vi "Snake.vi"(10 "Snake":dbl, 11 "Crab Degree":dbl) -> (0 "FR":dbl, 1 "FL":dbl, 2 "RR":dbl, 3 "RL":dbl)   [LabVIEW 2016]
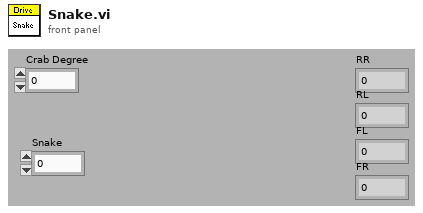
[diagram p1: front panel]
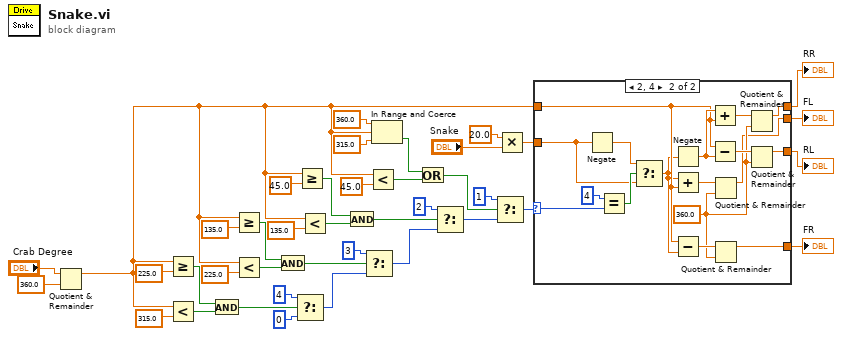
[diagram p0: block diagram]
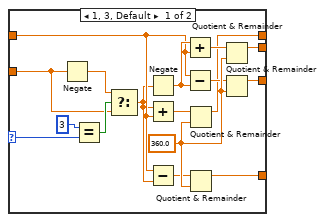
[diagram p2: hidden frame]
diagram:
  n1 = Quotient & Remainder(x="Crab Degree", y=360.0) -> (x-y*floor(x/y)=w1:dbl)  [unwired: 1 out]
  n2 = Greater Or Equal?(x=w1, y=225.0) -> (x >= y?=w18:bool)
  n3 = Less?(x=w1, y=315.0) -> (x < y?=w19:bool)
  n4 = And(x=w18, y=w19) -> (x .and. y?=w17:bool)
  n5 = Greater Or Equal?(x=w1, y=135.0) -> (x >= y?=w25:bool)
  n6 = Less?(x=w1, y=225.0) -> (x < y?=w24:bool)
  n7 = And(x=w25, y=w24) -> (x .and. y?=w11:bool)
  n8 = Select(t=4, s=w17, f=0) -> (s? t:f=w16:i32)
  n9 = Greater Or Equal?(x=w1, y=45.0) -> (x >= y?=w26:bool)
  n10 = Less?(x=w1, y=135.0) -> (x < y?=w27:bool)
  n11 = And(x=w26, y=w27) -> (x .and. y?=w12:bool)
  n12 = Select(t=3, s=w11, f=w16) -> (s? t:f=w15:i32)
  n13 = Less?(x=w1, y=45.0) -> (x < y?=w31:bool)
  n14 = In Range and Coerce(upper limit=360.0, x=w1, lower limit=315.0) -> (In Range?=w30:bool)  [unwired: 1 out]
  n15 = Or(x=w30, y=w31) -> (x .or. y?=w13:bool)
  n16 = Select(t=2, s=w12, f=w15) -> (s? t:f=w14:i32)
  n17 = Select(t=1, s=w13, f=w14) -> (s? t:f=w5:i32)
  n18 = Multiply(x=20.0, y="Snake") -> (x*y=w35:dbl)
  n19 = case shown="2, 4" w5 {
    selector: w5 -> [w46 w62]
    tunnel: [w48 w68] -> w40
    tunnel: [w49 w67] -> w39
    tunnel: [w47 w66] -> w38
    tunnel: [w50 w65] -> w37
    tunnel: w1 -> [w51 w64]
    tunnel: w35 -> [w42 w59]
    frame 1, 3, Default {
      w57 = 360.0 ("y")
      n20 = Negate(x=w42) -> (-x=w43:dbl)
      n21 = Equal?(x=3, y=w46) -> (x = y?=w44:bool)
      n22 = Select(t=w43, s=w44, f=w42) -> (s? t:f=w41:dbl)
      n23 = Negate(x=w41) -> (-x=w52:dbl)
      n24 = Add(x=w41, y=w51) -> (x+y=w55:dbl)
      n25 = Subtract(x=w51, y=w41) -> (x-y=w56:dbl)
      n26 = Add(x=w52, y=w51) -> (x+y=w53:dbl)
      n27 = Subtract(x=w51, y=w52) -> (x-y=w54:dbl)
      n28 = Quotient & Remainder(x=w55, y=w57) -> (x-y*floor(x/y)=w49:dbl)  [unwired: 1 out]
      n29 = Quotient & Remainder(x=w56, y=w57) -> (x-y*floor(x/y)=w47:dbl)  [unwired: 1 out]
      n30 = Quotient & Remainder(x=w53, y=w57) -> (x-y*floor(x/y)=w50:dbl)  [unwired: 1 out]
      n31 = Quotient & Remainder(x=w54, y=w57) -> (x-y*floor(x/y)=w48:dbl)  [unwired: 1 out]
    }
    frame 2, 4 {
      w69 = 360.0 ("y")
      n32 = Negate(x=w59) -> (-x=w60:dbl)
      n33 = Equal?(x=4, y=w62) -> (x = y?=w61:bool)
      n34 = Select(t=w60, s=w61, f=w59) -> (s? t:f=w58:dbl)
      n35 = Negate(x=w58) -> (-x=w74:dbl)
      n36 = Add(x=w58, y=w64) -> (x+y=w71:dbl)
      n37 = Subtract(x=w64, y=w58) -> (x-y=w70:dbl)
      n38 = Add(x=w74, y=w64) -> (x+y=w73:dbl)
      n39 = Subtract(x=w64, y=w74) -> (x-y=w72:dbl)
      n40 = Quotient & Remainder(x=w71, y=w69) -> (x-y*floor(x/y)=w65:dbl)  [unwired: 1 out]
      n41 = Quotient & Remainder(x=w70, y=w69) -> (x-y*floor(x/y)=w66:dbl)  [unwired: 1 out]
      n42 = Quotient & Remainder(x=w73, y=w69) -> (x-y*floor(x/y)=w67:dbl)  [unwired: 1 out]
      n43 = Quotient & Remainder(x=w72, y=w69) -> (x-y*floor(x/y)=w68:dbl)  [unwired: 1 out]
    }
  }
  "RR" <- w39
  "RL" <- w40
  "FL" <- w37
  "FR" <- w38
